vi "FeederSystem.vi"() -> ()   [LabVIEW 2025]
panel:
  out "FeederSystem/FeederRPM":dbl caption="Speed RPM" format="%12.1f"
  out "FeederSystem/FeederOutput":dbl caption="Motor Dmd" format="%11.2f"
  out "FeederSystem/FeederState":bool caption="Feeder On"
  # "FEEDER"
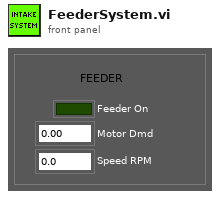
[diagram p1: front panel]
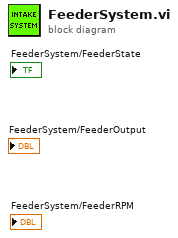
[diagram p0: block diagram]
diagram:
